vi "Configure Channel.vi"(0 "TDS 2000 in":refnum<class "TDS 2000.lvclass">, 1 "Vertical Scale (5.0 V)":dbl=5.0, 2 "Enable Channel (True)":bool=TRUE, 3 "Impedance (0: 1 MOhm)":i32(ring) items=["1 MOhm", "50 Ohm"], 5 "Cluster":T1={"Channel (0: Channel 1)"=0, "Vertical Coupling (1: DC)"=1, "Probe Attenuation (10: 10X)"=10, "Vertical Range (10.0 V/div)"=10.0, "Vertical Offset (0.0 divs)"=0.0, "Bandwidth (0: MAX Bandwidth)"=0} {"Bandwidth (0: MAX Bandwidth)" items=["MAX Bandwidth", "Unlimited"]; "Probe Attenuation (10: 10X)" items=["1"=1, "10"=10, "20"=20, "50"=50, "100"=100, "500"=500, "1000"=1000]; "Vertical Coupling (1: DC)" items=["AC", "DC", "Ground"]; "Channel (0: Channel 1)" items=["Channel 1", "Channel 2", "Channel 3", "Channel 4", "Math", "Reference A", "Reference B", "Reference C", "Reference D"]}, 11 "error in (no error)":errorcluster, 14 "Vertical Setting (1: Vertical Range)":i32(ring)=1 items=["Vertical Scale", "Vertical Range"]) -> (4 "TDS 2000 out":refnum<class "TDS 2000.lvclass">, 15 "error out":errorcluster)   [LabVIEW 2020, in "Oscilloscope.lvlib" / "TDS 2000.lvclass"]
uses:
  TDS 2000.lvclass
  C:/Users/ronad/Osciloscopio/Osciloscopio DQMH/Libraries/Oscilloscope/Clases/Osciloscopio/Osciloscopio.lvclass
  Osciloscopio/Osciloscopio.lvclass/Osciloscopio.ctl
  Osciloscopio/Read COM.vi
  Osciloscopio/Write COM.vi
  <instrlib>/Tektronix TDS 200 1000 2000 Series/Tektronix TDS 200 1000 2000 Series.lvlib
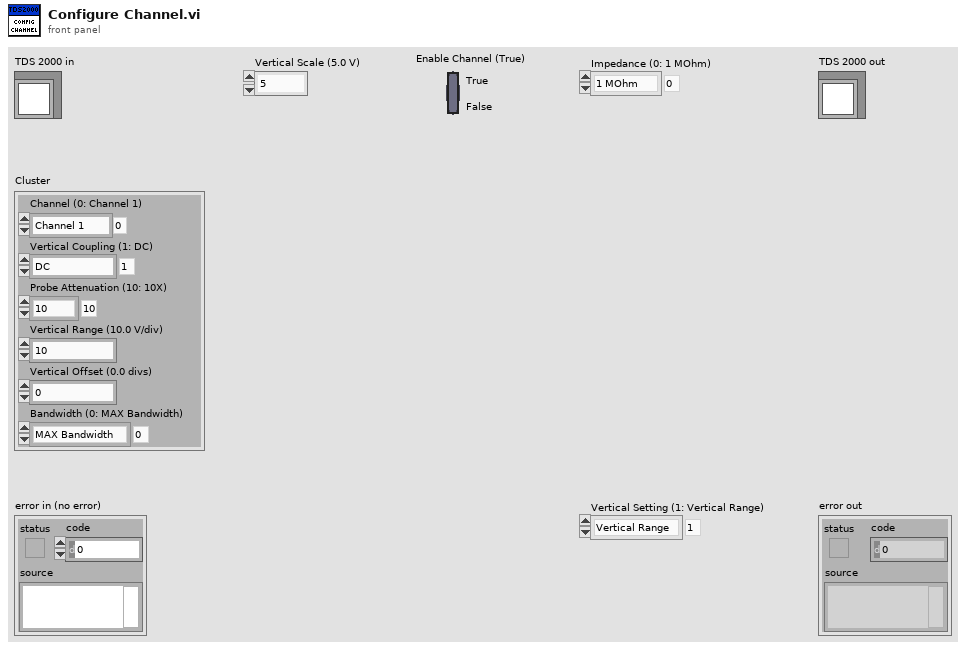
[diagram p1: front panel]
types:
  T1 = cluster{"Channel (0: Channel 1)":i32, "Vertical Coupling (1: DC)":i32, "Probe Attenuation (10: 10X)":i32, "Vertical Range (10.0 V/div)":dbl, "Vertical Offset (0.0 divs)":dbl, "Bandwidth (0: MAX Bandwidth)":i32}
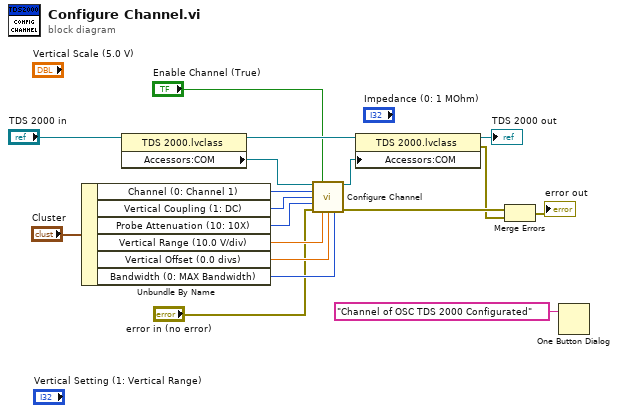
[diagram p0: block diagram]
diagram:
  n1 = Unbundle By Name("Cluster") -> ("Channel (0: Channel 1)"=w11:i32, "Vertical Coupling (1: DC)"=w10:i32, "Probe Attenuation (10: 10X)"=w9:i32, "Vertical Range (10.0 V/div)"=w8:dbl, "Vertical Offset (0.0 divs)"=w7:dbl, "Bandwidth (0: MAX Bandwidth)"=w6:i32)
  n2 = property class="TDS 2000.lvclass"(reference="TDS 2000 in") -> (reference out=w15:refnum<class "TDS 2000.lvclass">, "Accessors:COM"=w17:refnum<visa-resource-name>)  [unwired: 1 in, 1 out]
  n3 = call <instrlib>:"Configure Channel.vi"("VISA resource name"=w17, "Enable Channel (True)"="Enable Channel (True)", "Channel (0: Channel 1)"=w11, "Vertical Coupling (1: DC)"=w10, "Probe Attenuation (10: 10X)"=w9, "error in (no error)"="error in (no error)", "Vertical Range (10.0 V/div)"=w8, "Vertical Offset (0.0 divs)"=w7, "Bandwidth (0: MAX Bandwidth)"=w6) -> ("VISA resource name out"=w16:refnum<visa-resource-name>, "error out"=w5:errorcluster)  [unwired: 5 in]
  n4 = property class="TDS 2000.lvclass"(reference=w15, "Accessors:COM"=w16) -> (reference out=→"TDS 2000 out":refnum<class "TDS 2000.lvclass">, error out=w2:errorcluster)  [unwired: 1 in]
  n5 = Merge Errors(w5, w2) -> (→"error out":errorcluster)
  n6 = One Button Dialog(message="Channel of OSC TDS 2000 Configurated") -> ()  [unwired: 1 in, 1 out]
